vi "EncoderMake.vi"(9 "C":bool, 10 "B":bool, 11 "A":bool) -> (3 "Encoder Array":bool[](array[boolean]))   [LabVIEW 2018, in "kevLib2010.lvlib"]
uses:
  kevLib2010.lvlib
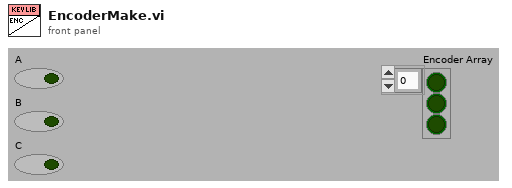
[diagram p1: front panel]
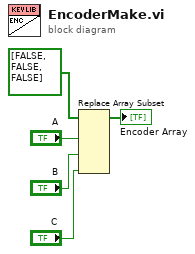
[diagram p0: block diagram]
diagram:
  n1 = Replace Array Subset(array=bool[] [FALSE, FALSE, FALSE], new element #1="A", new element #2="B", new element #3="C") -> (→"Encoder Array":bool[])  [unwired: 3 in]
